vi "MPS_Spectroscopy_Core.vi"(0 "EmptyBoreBaseline_Spec":dbl[](array[numeric])=array[21000 elements], 1 "ms delay":u32=25 format="%#.4p", 3 "Spec samples\nto crop":dbl=1000.0 format="%#_4p") -> (5 "Raw Measured":dbl[](array[numeric]), 6 "f0 Complex":cdb=-0.004151438219837607-0.0046789149193528995i, 7 "phase f1-f9":dbl[](array[numeric])=[-2.296530890286755, -0.4996795442572583, 2.13231335701235, -2.8305146270300687, -3.0644603787657894, -1.910517808964867, -1.4604887262767599, -1.4608770943170013, -0.49288277337997893] format="%#_4g", 8 "TF Corr Rx FFT Mag":cluster{"f0":dbl, "df":dbl, "magnitude":dbl[]}, 9 "TF units from loaded file":string, 10 "Spec Waveform Baseline Sub":waveform(dbl)={"t0"=timestamp(3728232981.5205336 s since 1904-01-01), "dt"=9.9999999999997e-07, "Y"=array[20000 elements], "attributes"=variant("NI_ChannelName"=variant(string "H1/ai7"), "NI_UnitDescription"=variant(string "Volts"))}, 11 "Drive IMon":waveform(dbl)(graph)={"t0"=timestamp(3728232981.5496345 s since 1904-01-01), "dt"=9.9999999999997e-07, "Y"=array[21000 elements], "attributes"=variant("NI_ChannelName"=variant(string "H1/ai4"), "NI_UnitDescription"=variant(string "Volts"))}, 12 "3f0 Complex":cdb=-1.808865307320394e-10+2.875482942470047e-10i, 13 "mag f1-f9":dbl[](array[numeric])=[0.006255132621749245, 5.349180742819057e-10, 3.3971158138137566e-10, 2.020645150662673e-11, 3.443682420408273e-11, 3.747219651257019e-11, 4.2635827797213496e-11, 3.5893791114801e-11, 3.560739858812373e-11] format="%#_4p", 14 "RX magnitude 3":dbl=3.3971158138137566e-10, 15 "Expected mT Spec Drive":dbl=0.03824103018872398 format="%#_4p", 16 "TF Corrected\nMagnetization over time":waveform(dbl)[](graph), 17 "Spec Time Domain":dbl[][](graph), 18 "Amps Drive Spec":dbl=0.058832354136498434 format="%#_4p", 19 "THD":dbl=1.5484776612982656 format="%#_6p")   [LabVIEW 2021]
uses:
  <vilib>/Analysis/4window.llb/windowTd.ctl
  <extravilib>/ChannelInstances/Tag-dbl/Write With Abort.vi
  MPS_global_variables.vi
  <extravilib>/ChannelInstances/Tag-dbl/Instantiate.vi
  <extravilib>/ChannelInstances/Tag-dbl/Endpoint.vi
  <vilib>/measure/maspectr.llb/FFT Spectrum (Mag-Phase) for 1 Chan.vi
  <vilib>/measure/matone.llb/Extract Single Tone Information 1 Chan.vi
  <extravilib>/ChannelInstances/Tag-dbl.lvlib
  <vilib>/measure/NI_MAPro.lvlib
  <vilib>/Analysis/NI_AALPro.lvlib
panel:
  out "dMdt":dbl[](graph)
  out "3f0 over time":dbl(graph)=3.3971158138137566e-10
  out "Drive IMon FFT":cluster{"f0":dbl, "df":dbl, "magnitude":dbl[]}(graph)={"f0"=0.0, "df"=47.61904761904904, "magnitude"=array[10500 elements]}
  out "detected amplitude\nDrive IMon":dbl=0.0003328133743989285 format="%.4p"
  out "Samples Per Acquisition":dbl=21000.0
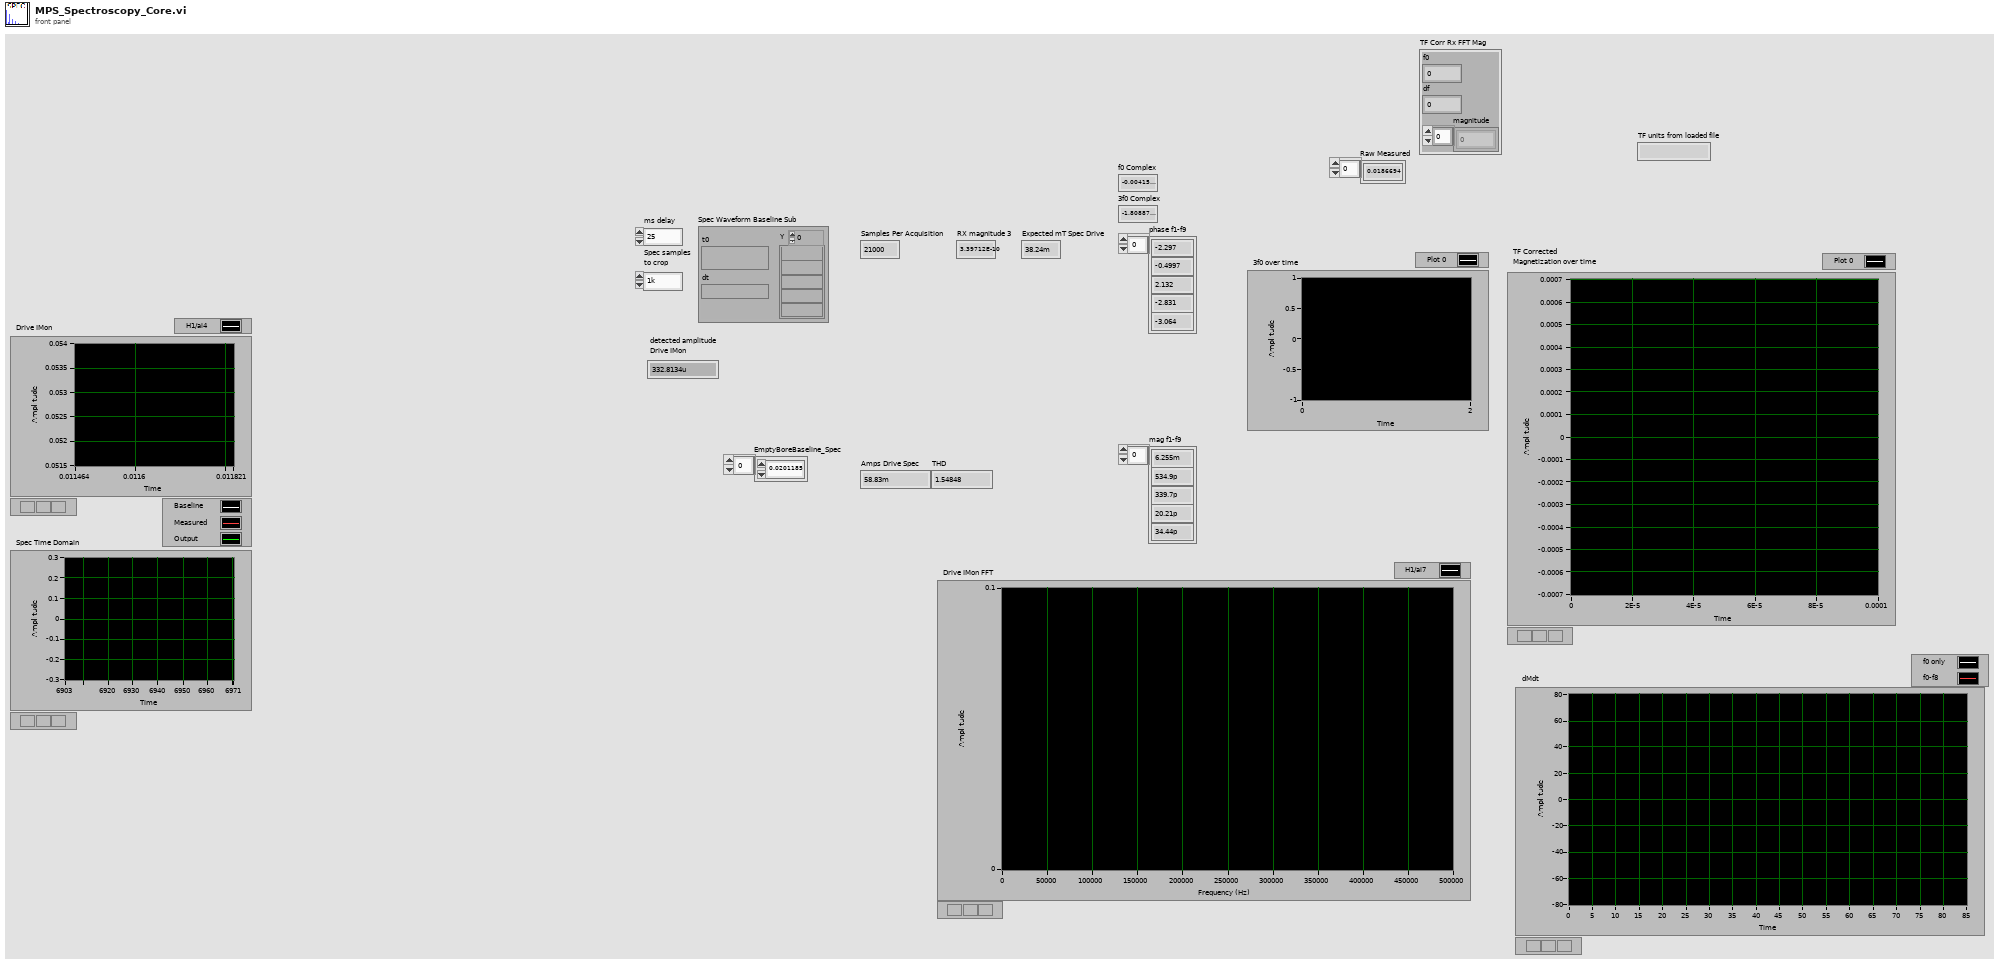
[diagram p1: front panel]
types:
  T1 = cluster{"sample rate":dbl, "Transmit frequency":dbl, "Transmit amplitude":dbl, "sample rate digital out":dbl, "TX cycles":i32, "sample rate DAQ1":dbl, "Receive frequency":dbl, "Receive range":dbl, "TX harmonics":dbl[]}
  T2 = typedef "NI_AALPro.lvlib/windowTd.ctl" = u32
  T3 = cluster{"sample rate":dbl, "Tx freq":dbl, "Tx amp":dbl, "Tx cycles\nSpectroscopy":dbl, "Bias amp":dbl, "Bias freq":dbl, "Receive range":dbl, "Bias Periods\nMagnetometry":dbl, "Tx Freq Division Factor":dbl, "Drive Periods per Bias":dbl, "TX harmonics":dbl[]}
  T4 = typedef "Tag-dbl.lvlib/))Channel.ctl" = refnum<queue>
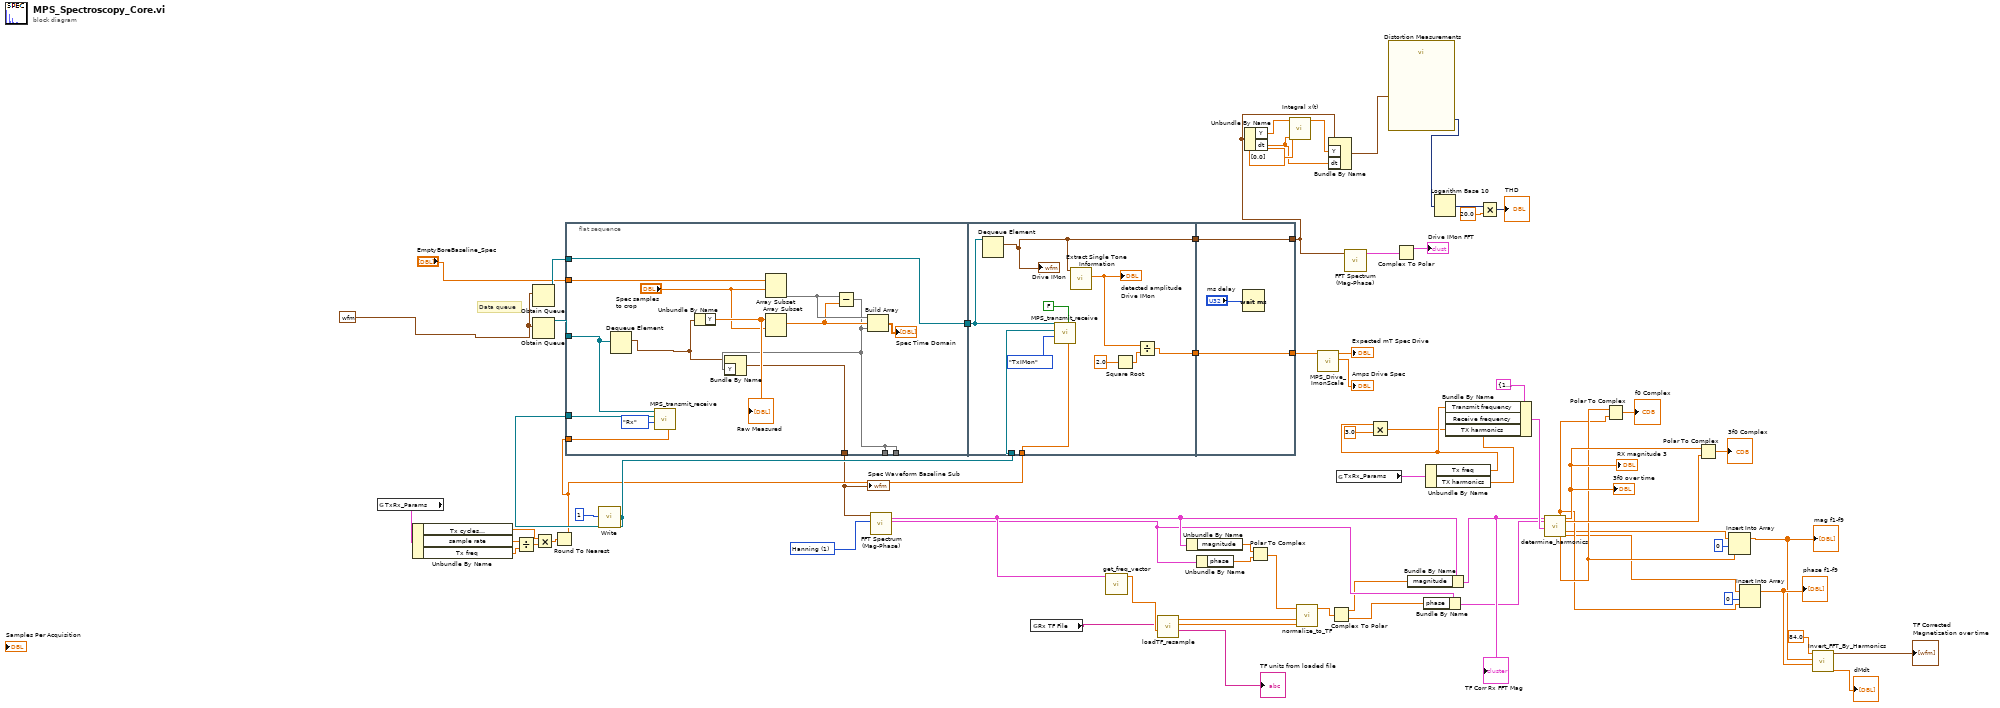
[diagram p0: block diagram]
diagram:
  w63 = T2 1 items=["Rectangle"=0, "Hanning"=1, "Hamming"=2, "Blackman-Harris"=3, "Exact Blackman"=4, "Blackman"=5, "Flat Top"=6, "4 Term B-Harris "=7, "7 Term B-Harris"=8, "Low Sidelobe"=9, "Blackman Nuttall"=11, "Triangle"=30, "Bartlett-Hanning"=31, "Bohman"=32, "Parzen"=33, "Welch"=34, "Kaiser"=60, "Dolph-Chebyshev"=61, "Gaussian"=62] ("window")
  w7 = waveform(dbl) {"t0"=timestamp(0 s since 1904-01-01), "dt"=1.0, "Y"=[]} ("Waveform")
  # "Data queue"
  n1 = global read "MPS_global_variables.vi" "TxRx_Params"() -> (w62:T3)
  n2 = Unbundle By Name(w62) -> ("Tx cycles\nSpectroscopy"=w58:dbl, "sample rate"=w61:dbl, "Tx freq"=w60:dbl)
  n3 = Divide(x=w61, y=w60) -> (x/y=w59:dbl)
  n4 = Obtain Queue(element data type=w7) -> (queue out=w64:refnum<queue>)  [unwired: 4 in, 2 out]
  n5 = Obtain Queue(element data type=w7) -> (queue out=w65:refnum<queue>)  [unwired: 4 in, 2 out]
  n6 = Multiply(x=w58, y=w59) -> (x*y=w57:dbl)
  n7 = Round To Nearest(number=w57) -> (nearest integer value=w56:dbl)
  n8 = flat-sequence {
    tunnel: w65 -> [w83]
    tunnel: [w82] -> w70
    tunnel: w66 -> [w84]
    tunnel: w64 -> [w82]
    tunnel: w56 -> [w81]
    tunnel: [w77] -> w48
    tunnel: [w74] -> _
    tunnel: [w74] -> _
    tunnel: "EmptyBoreBaseline_Spec" -> [w73]
    tunnel: w70 -> [w92]
    tunnel: w66 -> [w94]
    tunnel: w56 -> [w93]
    tunnel: [w89] -> w69
    tunnel: [w85] -> w68
    tunnel: [w97] -> w2
    tunnel: w69 -> [w97]
    tunnel: w68 -> [w95]
    tunnel: [w95] -> w40
    frame #0 {
      n9 = Dequeue Element(queue=w83) -> (element=w71:waveform(dbl))  [unwired: 2 in, 3 out]
      n10 = call "MPS_transmit_receive.vi"("samples per readout"=w81, "InputChans"=enum16{"Rx", "BiasIMon", "TxIMon", "BMon"}."Rx", "channel input for max readouts"=w84, "Measurement Queue"=w83) -> ()  [unwired: 8 in]
      n11 = Unbundle By Name(w71) -> ("Y"=w79:dbl[])
      "Raw Measured" <- w79
      n12 = Array Subset(array=w73, index="Spec samples\nto crop") -> (w76:dbl[])  [unwired: 1 in]
      n13 = Array Subset(array=w79, index="Spec samples\nto crop") -> (w75:dbl[])  [unwired: 1 in]
      n14 = Subtract(x=w76, y=w75) -> (x-y=w74:dbl[])
      n15 = Bundle By Name(cluster=w71, "Y"=w74) -> (w77:waveform(dbl))
      n16 = Build Array(w76, w75, w74) -> (→"Spec Time Domain":dbl[][])
    }
    frame #1 {
      n17 = Dequeue Element(queue=w92) -> (element=w89:waveform(dbl))  [unwired: 2 in, 3 out]
      "Drive IMon" <- w89
      n18 = call "MPS_transmit_receive.vi"("samples per readout"=w93, "Use Bias?"=FALSE, "InputChans"=enum16{"Rx", "BiasIMon", "TxIMon", "BMon"}."TxIMon", "channel input for max readouts"=w94, "Measurement Queue"=w92) -> ()  [unwired: 7 in]
      n19 = call-poly <vilib>:"Extract Single Tone Information.vi"("time signal in"=w89) -> ("detected amplitude"=w87:dbl)  [unwired: 5 in, 5 out]
      "detected amplitude\nDrive IMon" <- w87
      n20 = Square Root(x=2.0) -> (sqrt(x)=w88:dbl)
      n21 = Divide(x=w87, y=w88) -> (x/y=w85:dbl)
    }
    frame #2 {
      n22 = Wait (ms)(milliseconds to wait="ms delay") -> ()  [unwired: 1 out]
    }
  }
  n23 = call <extravilib>:"Write.vi"("element"=1 ("number of readouts")) -> ("channel"=w66:T4)  [unwired: 1 out]
  n24 = call-poly <vilib>:"FFT Spectrum (Mag-Phase).vi"("window"=w63, "time signal"=w48) -> ("phase"=w22:cluster{"f0":dbl, "df":dbl, "phase":dbl[]}, "magnitude"=w23:cluster{"f0":dbl, "df":dbl, "magnitude":dbl[]})  [unwired: 5 in, 3 out]
  n25 = global read "MPS_global_variables.vi" "Rx TF File"() -> (w10:string)
  n26 = call "get_freq_vector.vi"("FFT magnitude"=w23) -> ("Freq array"=w27:dbl[])  [unwired: 10 in]
  n27 = call "loadTF_resample.vi"("desired freqs"=w27, "mat file name"=w10) -> ("TF units from loaded file"=→"TF units from loaded file":string, "output TF phase"=w29:dbl[], "output TF mag"=w28:dbl[])  [unwired: 7 in]
  n28 = Unbundle By Name(w23) -> ("magnitude"=w26:dbl[])
  n29 = Unbundle By Name(w22) -> ("phase"=w25:dbl[])
  n30 = Unbundle By Name(w2) -> ("Y"=w6:dbl[], "dt"=w4:dbl)
  n31 = Polar To Complex(1:w25, 2:w26) -> (0:w24:cdb[])
  n32 = call <vilib>:"Integral x(t).vi"("dt"=w4, "Initial Condition"=dbl[] [0.0], "X"=w6) -> ("Integral X"=w3:dbl[])  [unwired: 7 in, 1 out]
  n33 = call "normalize_to_TF.vi"("TF phase"=w29, "TF mag"=w28, "signal (can be complex)"=w24) -> ("signal normalized to TF (can be complex)"=w17:cdb[])  [unwired: 8 in]
  n34 = call "MPS_Drive_ImonScale.vi"("Drive IMon FFT Mag RMS"=w40) -> ("Amps Drive Peak"=→"Amps Drive Spec":dbl, "Expected mT Peak"=→"Expected mT Spec Drive":dbl)  [unwired: 9 in]
  n35 = Bundle By Name(cluster=w2, "Y"=w3, "dt"=w4) -> (w1:waveform(dbl))
  n36 = Complex To Polar(r * e^(i*theta)=w17) -> (r=w21:dbl[], theta=w20:dbl[])
  n37 = global read "MPS_global_variables.vi" "TxRx_Params"() -> (w53:T3)
  n38 = call-poly <vilib>:"FFT Spectrum (Mag-Phase).vi"("time signal"=w2) -> ("magnitude"=w52:cluster{"f0":dbl, "df":dbl, "magnitude":dbl[]})  [unwired: 6 in, 4 out]
  n39 = call "Distortion Measurements"("Signals"=w1) -> ("THD"=w47:dynamicdata)  [unwired: 8 in, 2 out]
  n40 = Complex To Polar(r * e^(i*theta)=w52) -> (r=→"Drive IMon FFT":cluster{"f0":dbl, "df":dbl, "magnitude":dbl[]})  [unwired: 1 out]
  n41 = Bundle By Name(cluster=w23, "magnitude"=w21) -> (w19:cluster{"f0":dbl, "df":dbl, "magnitude":dbl[]})
  "TF Corr Rx FFT Mag" <- w19
  n42 = Bundle By Name(cluster=w22, "phase"=w20) -> (w18:cluster{"f0":dbl, "df":dbl, "phase":dbl[]})
  n43 = Unbundle By Name(w53) -> ("Tx freq"=w42:dbl, "TX harmonics"=w39:dbl[])
  n44 = Multiply(x=w42, y=3.0) -> (x*y=w41:dbl)
  n45 = Logarithm Base 10(1:w47) -> (0:w45:dynamicdata)
  n46 = Bundle By Name(cluster=T1 {"sample rate"=1000000.0, "Transmit frequency"=25000.0, "Transmit amplitude"=1.577, "sample rate digital out"=40000.0, "TX cycles"=600, "sample rate DAQ1"=1000000.0, "Receive frequency"=75000.0, "Receive range"=1.0, "TX harmonics"=[50000.0, 75000.0, 100000.0, 125000.0, 150000.0, 175000.0, 200000.0, 225000.0]} ("TxRxParams"), "Transmit frequency"=w42, "Receive frequency"=w41, "TX harmonics"=w39) -> (w51:T1)
  n47 = Multiply(x=w45, y=20.0) -> (x*y=→"THD":dynamicdata)
  n48 = call "determine_harmonics.vi"("FFT magnitude"=w19, "FFT phase"=w18, "TxRxParams"=w51) -> ("f0 phase"=w30:dbl, "f0 mag"=w31:dbl, "RX magnitude"=w35:dbl, "RX phase"=w36:dbl, "mag f2-f9"=w14:dbl[], "phase f2-f9"=w15:dbl[])  [unwired: 11 in]
  "RX magnitude 3" <- w35
  "3f0 over time" <- w35
  n49 = Polar To Complex(1:w30, 2:w31) -> (0:→"f0 Complex":cdb)
  n50 = Polar To Complex(1:w36, 2:w35) -> (0:→"3f0 Complex":cdb)
  n51 = Insert Into Array(array=w14, index=0, new element=w31) -> (w11:dbl[])
  "mag f1-f9" <- w11
  n52 = Insert Into Array(array=w15, index=0, new element=w30) -> (w12:dbl[])
  "phase f1-f9" <- w12
  n53 = call "Invert_FFT_By_Harmonics.vi"("phase f1-f9"=w12, "mag f1-f9"=w11, "Num Samp"=84.0) -> ("dMdt"=→"dMdt":dbl[], "Waveform Graph"=→"TF Corrected\nMagnetization over time":waveform(dbl)[])  [unwired: 6 in, 1 out]
  "Spec Waveform Baseline Sub" <- w48
